vi "Falling Edge Detect.vi"(4 "Input":bool) -> (1 "Pulse":bool)   [LabVIEW 2013]
doc: "This VI generates a single-cycle pulse each time there is a high-to-low transition on the input signal. This makes it easy to detect falling edges on signals."
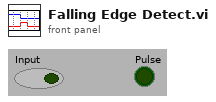
[diagram p1: front panel]
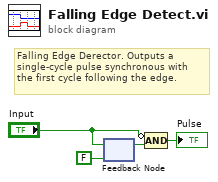
[diagram p0: block diagram]
diagram:
  # "Falling Edge Derector. Outputs a\nsingle-cycle pulse synchronous with\nthe first cycle following the edge."
  n1 = feedback-in #1("Input") -> ()
  n2 = feedback #1(FALSE ("FV")) -> (w3:bool)
  n3 = Compound Arithmetic op=AND(invert "Input", w3) -> (→"Pulse":bool)
